vi "Lorentzian phase test.vi"(3 "output control":T1, 4 "data":variant, 5 "X":dbl[](array[numeric]), 6 "a":dbl[](array[numeric])) -> (0 "error out":errorcluster, 1 "f'(X,a)":dbl[][](array[numeric]), 2 "f(X,a)":dbl[](array[numeric]))   [LabVIEW 2016]
doc: "Sum of three Gaussians, plus DC offset."
uses:
  <vilib>/gmath/NumericalOptimization/LM_output select.ctl
  <vilib>/gmath/NI_Gmath.lvlib
panel:
  out "Waveform Graph":dbl[](graph)
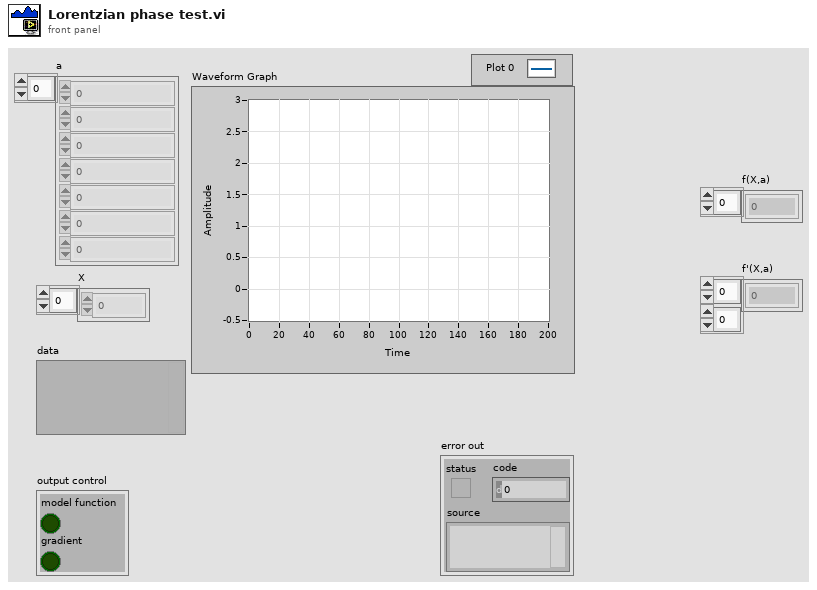
[diagram p1: front panel]
types:
  T1 = typedef "NI_Gmath.lvlib/LM_output select.ctl" = cluster{"model function":bool, "gradient":bool}
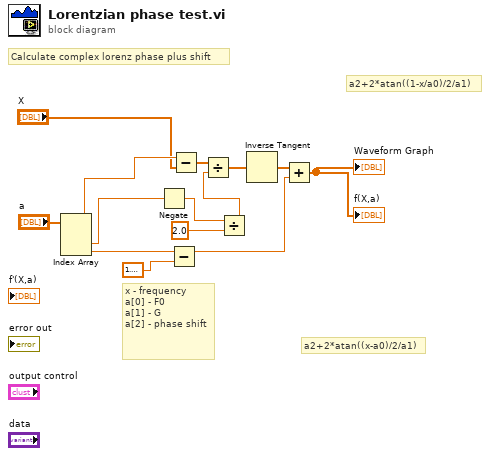
[diagram p0: block diagram]
diagram:
  # "a2+2*atan((x-a0)/2/a1)"
  # "x - frequency\na[0] - F0\na[1] - G\na[2] - phase shift"
  # "a2+2*atan((1-x/a0)/2/a1)"
  # "Calculate complex lorenz phase plus shift"
  n1 = Index Array(array="a") -> (element #1=w7:dbl, element #2=w12:dbl, element #3=w10:dbl)  [unwired: 3 in]
  n2 = Negate(x=w12) -> (-x=w2:dbl)
  n3 = Subtract(x=w10, y=1.5707963267948966) -> (x-y=w5:dbl)
  n4 = Subtract(x=w7, y="X") -> (x-y=w13:dbl[])
  n5 = Divide(x=w2, y=2.0) -> (x/y=w3:dbl)
  n6 = Divide(x=w13, y=w3) -> (x/y=w11:dbl[])
  n7 = Inverse Tangent(1:w11) -> (0:w9:dbl[])
  n8 = Add(x=w9, y=w5) -> (x+y=→"f(X,a)" →"Waveform Graph":dbl[])
